vi "Actor Core.vi"(8 "error in":errorcluster, 11 "UDP Service in":refnum<class "UDP Service.lvclass">) -> (0 "error out":errorcluster, 3 "Actor out":refnum<class "Actor.lvclass">)   [LabVIEW 2016, in "Assert API Components.lvlib" / "UDP Service.lvlib" / "UDP Service.lvclass"]
doc: "(<B>Filename</B>: Actor Framework.lvlib:Actor.lvclass:Actor Core.vi)\n\nReceives messages to the actor, reacts to them, and initiates any error handling that may shut the actor down.\n\nDescendant classes may override this VI to append parallel tasks for the actor to complete while it handles messages. Overrides use the Call Parent Method node."
uses:
  UDP Service.lvclass
  D:/Work/Projects/Actor_Assert_API/Base UI Actor/Base UI Actor/Base UI Actor.lvclass
  C:/Program Files (x86)/National Instruments/LabVIEW 2016/vi.lib/ActorFramework/Actor/Actor.lvclass
  <vilib>/ActorFramework/Actor/Actor.lvclass
  <vilib>/ActorFramework/Actor/Actor.lvclass/Actor.ctl
  Base UI Actor/Base UI Actor/Base UI Actor.lvclass/Base UI Actor.ctl
  UDP Service.lvclass/UDP Service.ctl
  Main Display/Main Display Messages/New Assert Message Msg/New Assert Message Msg.lvclass/New Assert Message Msg.ctl
  <vilib>/ActorFramework/Message Enqueuer/Message Enqueuer.lvclass/Message Enqueuer.ctl
  <vilib>/ActorFramework/Message Enqueuer/Enqueue.vi
  Main Display/Main Display Messages/New Assert Message Msg/New Assert Message Msg.lvclass
  C:/Program Files (x86)/National Instruments/LabVIEW 2016/vi.lib/ActorFramework/Message/Message.lvclass
  <vilib>/Utility/LVClass/Get LV Class Name.vi
  <resource>/AFDebug/Generate Trace for Message.vi
  <vilib>/ActorFramework/Message Priority Queue/Priority Enqueue.vi
  Base UI Actor/Base UI Actor/Base UI Actor.lvclass
panel:
  out "IP Address":string
  out "Service Name":string
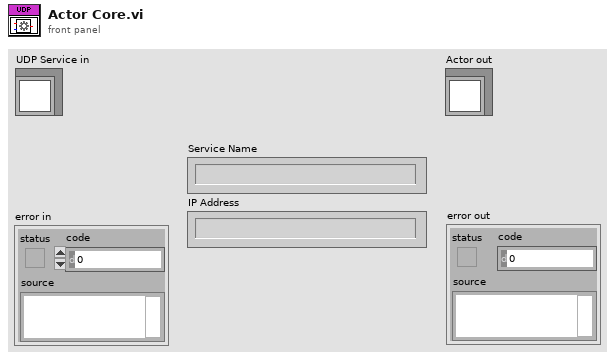
[diagram p1: front panel]
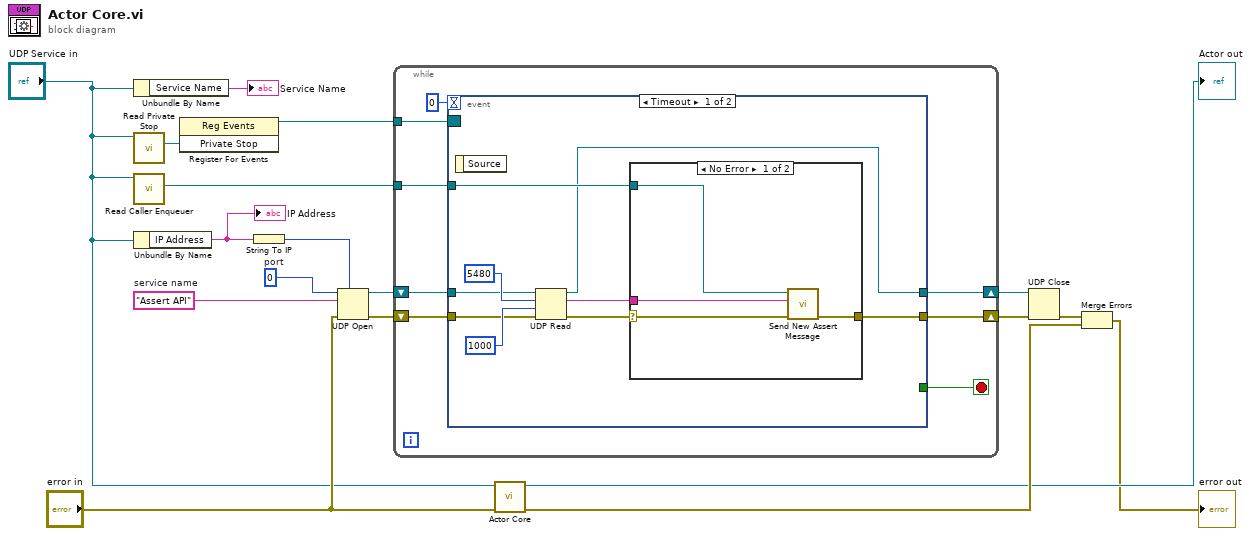
[diagram p0: block diagram]
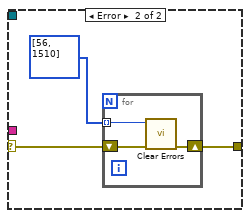
[diagram p2: hidden frame]
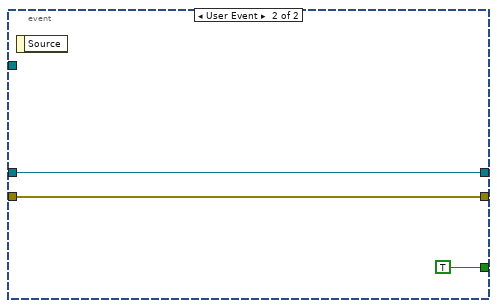
[diagram p3: hidden frame]
diagram:
  w12 = "Assert API"  # service name
  w11 = u16 0  # port
  n1 = Unbundle By Name("UDP Service in") -> ("Service Name"=→"Service Name":string)
  n2 = call "Read Private Stop.vi"("Base UI Actor in"="UDP Service in") -> ("Private Stop"=w16:refnum<user-event>)  [unwired: 10 in]
  n3 = call <vilib>:"Read Caller Enqueuer.vi"("Actor"="UDP Service in") -> ("Caller Enqueuer"=w7:refnum<class "Message Enqueuer.lvclass">)  [unwired: 10 in]
  n4 = Unbundle By Name("UDP Service in") -> ("IP Address"=w1:string)
  "IP Address" <- w1
  n5 = register-events(w16) -> (reference out=w15:refnum<event-registration>)  [unwired: 2 in, 1 out]
  n6 = String To IP(1:w1) -> (0:w13:u32)
  n7 = UDP Open(7:w13, 8:"error in", 10:w12, 11:w11) -> (port=w9:refnum<k16>, 0:w8:errorcluster)  [unwired: 1 in, 1 out]
  n8 = while {
    tunnel: w15 -> [w26]
    tunnel: w7 -> [w21]
    shift-right: [w19] -> w3
    shift-left: w9 -> [w23]
    shift-right: [w20] -> w5
    shift-left: w8 -> [w22]
    stop <- w24 stop-if-true
    n9 = event shown="[0] Timeout" {
      selector: w26 -> [_ _]
      dyn-events: _ -> [_ _]
      timeout: 0 -> [_ _]
      tunnel: [_ TRUE] -> w24
      tunnel: w23 -> [w31 w46]
      tunnel: w22 -> [w30 w47]
      tunnel: w21 -> [w29 _]
      tunnel: [w28 w47] -> w20
      tunnel: [w27 w46] -> w19
      event Timeout {
        n10 = event-data() -> ()  [unwired: 1 in, 1 out]
        n11 = UDP Read(connection ID=w31, max size (548)=5480, timeout ms (25000)=1000, 8:w30) -> (data out=w33:string, error out=w32:errorcluster, 3:w27:refnum<k16>)  [unwired: 2 out]
        n12 = case shown="No Error" w32 {
          selector: w32 -> [w38 w41]
          tunnel: [w39 w40] -> w28
          tunnel: w33 -> [w37 _]
          tunnel: w29 -> [w36 _]
          frame No Error {
            n13 = call "Send New Assert Message.vi"("error in (no error)"=w38, "Assert Message"=w37, "Message Enqueuer"=w36) -> ("error out"=w39:errorcluster)  [unwired: 7 in, 1 out]
          }
          frame Error {
            n14 = for {
              tunnel: i32[] [56, 1510] ("specific error code to clear (0: all)") -> [w45] mode=indexing
              shift-right: [w43] -> w40
              shift-left: w41 -> [w44]
              n15 = call <vilib>:"Clear Errors.vi"("error in (no error)"=w44, "specific error code to clear (0: all)"=w45) -> ("error out"=w43:errorcluster)  [unwired: 4 in, 1 out]
            }
          }
        }
      }
      event User Event {
        n16 = event-data() -> ()  [unwired: 1 in, 1 out]
      }
    }
  }
  n17 = call-parent "Actor Core.vi"("error in"="error in", "Actor in"="UDP Service in") -> ("error out"=w18:errorcluster, "Actor out"=→"Actor out":refnum<class "Actor.lvclass">)  [unwired: 8 in]
  n18 = UDP Close(connection ID=w3, 8:w5) -> (error out=w4:errorcluster)  [unwired: 1 out]
  n19 = Merge Errors(w4, w18) -> (→"error out":errorcluster)
